vi "NS master_Create.vi"(8 "error in (no error)":errorcluster, 10 "ID":string, 11 "reference in":refnum<class "NS master.lvclass">) -> (0 "error out":errorcluster, 3 "reference out":refnum<class "NS master.lvclass">)   [LabVIEW 2019, in "CommandResponse communication.lvlib" / "NS master.lvclass"]
doc: "Constructor."
uses:
  NS master.lvclass
  C:/Program Files/National Instruments/LabVIEW 2019/vi.lib/addons/_AddQ/G#Object/G#Object.lvclass
  <vilib>/addons/_AddQ/G#Object/utils/G#Object_CreateMethod.ctl
  <vilib>/addons/_AddQ/G#Object/G#Object.lvclass
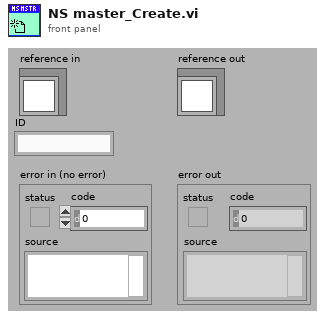
[diagram p1: front panel]
types:
  T1 = typedef "G#Object.lvclass/G#Object_CreateMethod.ctl" = enum16{"Create", "Create or look up existing", "Look up existing"}
  T2 = typedef "CommandResponse communication.lvlib/NS master.lvclass/ObjectAttributesRef.ctl" = refnum<data-value>
  T3 = typedef "CommandResponse communication.lvlib/NS master.lvclass/ObjectAttributes.ctl" = cluster{"connected":bool, "stop":bool, "ID":string, "command wr":refnum<k21>, "response rd":refnum<k21>, "data rd":refnum<k21>, "slave ip":string, "slave id":string}
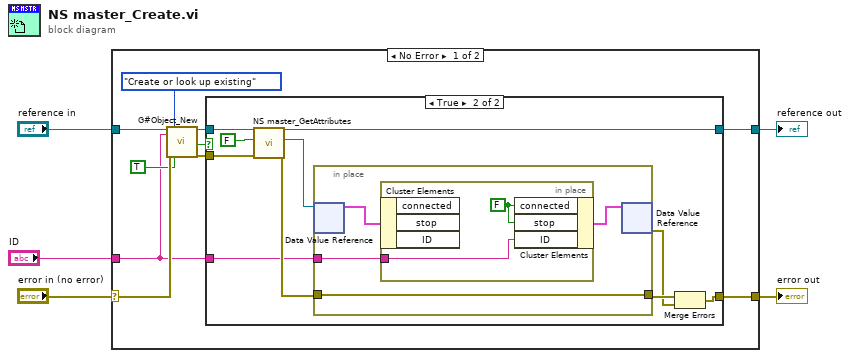
[diagram p0: block diagram]
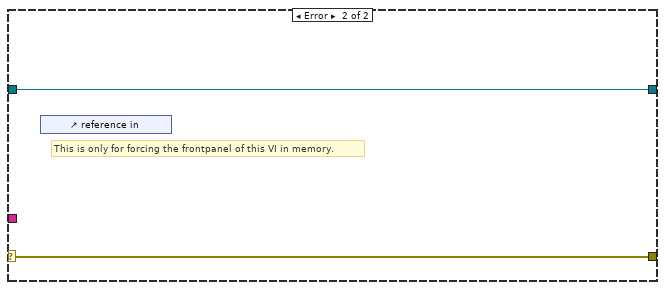
[diagram p3: hidden frame]
diagram:
  n1 = case shown="No Error" "error in (no error)" {
    selector: "error in (no error)" -> [w14 w35]
    tunnel: [w13 w35] -> w4
    tunnel: [w10 w34] -> w2
    tunnel: "reference in" -> [w15 w34]
    tunnel: "ID" -> [w8 _]
    frame No Error {
      n2 = call <vilib>:"G#Object_New.vi"("reference in"=w15, "object name"=w8, "error in (no error)"=w14, "create method"=G#Object_CreateMethod."Create or look up existing", "user counter (T)?"=TRUE ("User Counter")) -> ("reference out"=w11:refnum<class "NS master.lvclass">, "created new?"=w7:bool, "error out"=w9:errorcluster)  [unwired: 12 in]
      n3 = case shown="True" w7 {
        tunnel: [w16 w27] -> w13
        tunnel: w11 -> [w17 w24]
        tunnel: [w17 w23] -> w10
        tunnel: w9 -> [w16 w22]
        tunnel: w8 -> [_ w18]
        frame False {
        }
        frame True {
          n4 = call "NS master_GetAttributes.vi"("error in (no error)"=w22, "return data? (T)"=FALSE ("return data"), "reference in"=w24) -> ("error out"=w21:errorcluster, "attributes ref"=w20:T2, "reference out"=w23:refnum<class "NS master.lvclass">)  [unwired: 5 in, 1 out]
          n5 = in-place {
            in-place-border: w21 -> [w29]
            in-place-border: [w29] -> w26
            in-place-border: w18 -> [w28]
            n6 = in-place-dvr #1(w20) -> (w30:T3)  [unwired: 1 out]
            n7 = in-place {
              in-place-border: w28 -> [w32]
              w33 = FALSE ("connected")
              n8 = in-place-cluster #2(w30) -> ()  [unwired: 3 out]
              n9 = in-place-cluster #2("connected"=w33, "stop"=w33, "ID"=w32) -> (w31:T3)
            }
            n10 = in-place-dvr #1(w31) -> (w25:errorcluster)  [unwired: 1 out]
          }
          n11 = Merge Errors(w26, w25) -> (w27:errorcluster)
        }
      }
    }
    frame Error {
      # "This is only for forcing the frontpanel of this VI in memory."
      n12 = control-ref of="reference in"() -> ()  [unwired: 1 out]
    }
  }
  "error out" <- w4
  "reference out" <- w2
